vi "Revision Query.vi"(8 "error in (no error)":errorcluster, 11 "CS++DeviceActor in":refnum<class "CS++DeviceActor.lvclass">) -> (0 "error out":errorcluster, 1 "Firmware Revision":string, 2 "Driver Revision":string, 3 "CS++DeviceActor out":refnum<class "CS++DeviceActor.lvclass">)   [LabVIEW 2012, in "CS++DeviceActor.lvlib" / "CS++DeviceActor.lvclass"]
uses:
  CS++DeviceActor.lvclass
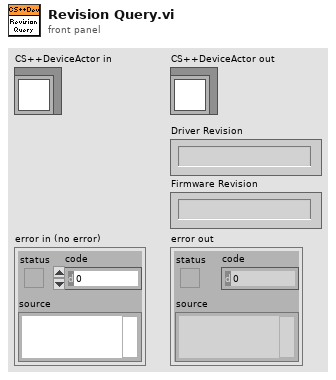
[diagram p1: front panel]
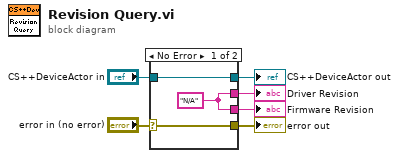
[diagram p0: block diagram]
diagram:
  n1 = case shown="No Error" "error in (no error)" {
    selector: "error in (no error)" -> [w8 w11]
    tunnel: [w8 w11] -> w5
    tunnel: [w9 w10] -> w3
    tunnel: "CS++DeviceActor in" -> [w9 w10]
    tunnel: [w7 _] -> w2
    tunnel: [w7 _] -> w1
    frame No Error {
      w7 = "N/A"
    }
    frame Error {
    }
  }
  "error out" <- w5
  "CS++DeviceActor out" <- w3
  "Driver Revision" <- w2
  "Firmware Revision" <- w1
